vi "S2C_M2p5942_Proc_CallAcquire.vi"(7 "Command":string, 8 "Error In":errorcluster, 11 "Data":T1) -> (0 "Error Out":errorcluster)   [LabVIEW 2024]
uses:
  S2C_M2p5942_Proc_Globals.vi
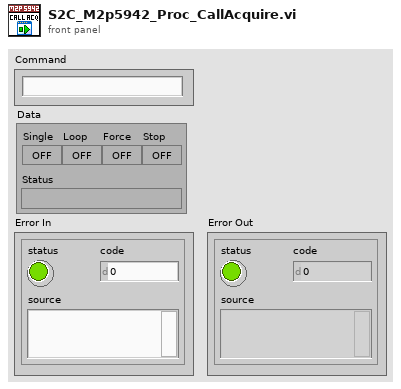
[diagram p1: front panel]
types:
  T1 = cluster{"Single":bool, "Loop":bool, "Force":bool, "Status":string, "Stop":bool}
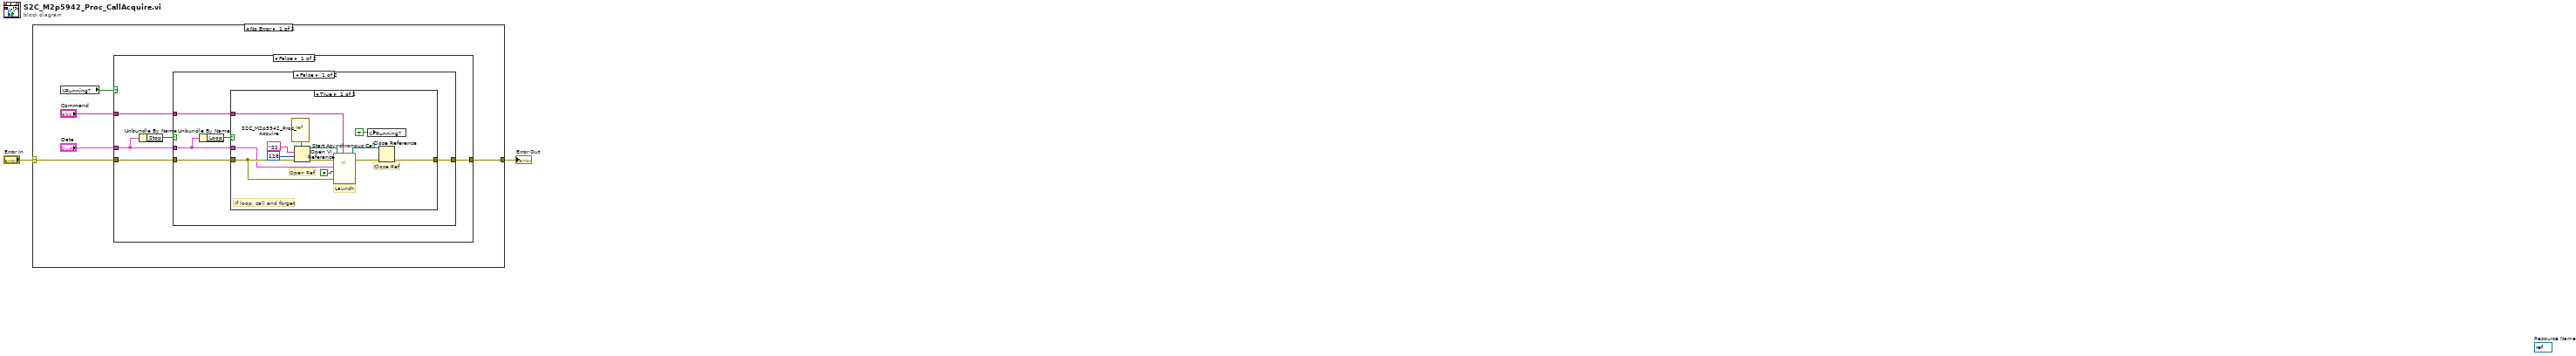
[diagram p0: block diagram]
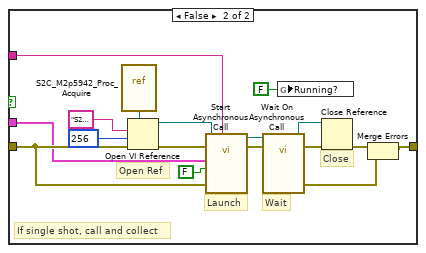
[diagram p2: hidden frame]
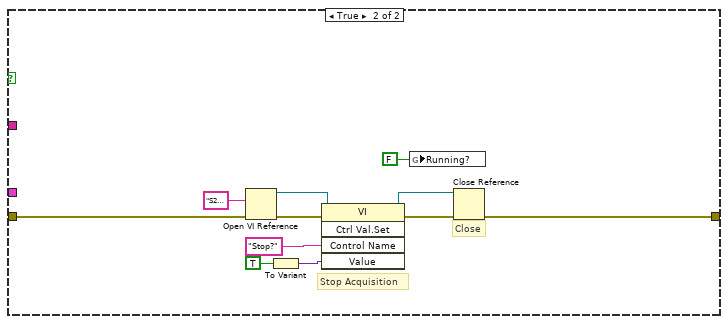
[diagram p4: hidden frame]
diagram:
  (unwired) refnum<visa-resource-name> refnum  # Resource Name
  n1 = case shown="No Error" "Error In" {
    selector: "Error In" -> [w7 w60]
    tunnel: [w6 w60] -> w1
    frame No Error {
      n2 = global read "S2C_M2p5942_Proc_Globals.vi" "Running?"() -> (w3:bool)
      n3 = case shown="False" w3 {
        tunnel: w7 -> [w12 w59]
        tunnel: [w11 w49] -> w6
        tunnel: "Command" -> [w10 _]
        tunnel: "Data" -> [w9 _]
        frame False {
          n4 = Unbundle By Name(w9) -> ("Stop"=w8:bool)
          n5 = case shown="False" w8 {
            tunnel: w12 -> [w17 w48]
            tunnel: [w16 w48] -> w11
            tunnel: w10 -> [w15 _]
            tunnel: w9 -> [w13 _]
            frame False {
              n6 = Unbundle By Name(w13) -> ("Loop"=w14:bool)
              n7 = case shown="True" w14 {
                tunnel: w15 -> [w24 w41]
                tunnel: w17 -> [w23 w40]
                tunnel: [w22 w35] -> w16
                tunnel: w13 -> [w21 w39]
                frame True {
                  # "If loop, call and forget"
                  # "Close Ref"
                  # "Launch"
                  # "Open Ref"
                  n8 = vi-ref "S2C_M2p5942_Proc_Acquire.vi"() -> (w29:refnum<vi>)
                  n9 = Open VI Reference(type specifier VI Refnum (for type only)=w29, vi path="S2C_M2p5942_Proc_Acquire.vi", options=128, error in (no error)=w23) -> (vi reference=w27:refnum<vi>, error out=w28:errorcluster)  [unwired: 2 in]
                  n10 = call-by-ref "Start Asynchronous Call"(reference=w27, error in=w28, "Command"=w24, "Error In"=w23, "Stop?"=FALSE, "Data"=w21) -> (reference out=w20:refnum<vi>, error out=w30:errorcluster)  [unwired: 7 in, 1 out]
                  n11 = global write "S2C_M2p5942_Proc_Globals.vi" "Running?"(TRUE ("Running?")) -> ()
                  n12 = Close Reference(reference=w20, error in (no error)=w30) -> (error out=w22:errorcluster)
                }
                frame False {
                  # "If single shot, call and collect"
                  # "Wait"
                  # "Close"
                  # "Launch"
                  # "Open Ref"
                  n13 = vi-ref "S2C_M2p5942_Proc_Acquire.vi"() -> (w46:refnum<vi>)
                  n14 = Open VI Reference(type specifier VI Refnum (for type only)=w46, vi path="S2C_M2p5942_Proc_Acquire.vi", options=256, error in (no error)=w40) -> (vi reference=w44:refnum<vi>, error out=w45:errorcluster)  [unwired: 2 in]
                  n15 = call-by-ref "Start Asynchronous Call"(reference=w44, error in=w45, "Command"=w41, "Error In"=w40, "Stop?"=FALSE, "Data"=w39) -> (reference out=w38:refnum<vi>, error out=w47:errorcluster)  [unwired: 7 in, 1 out]
                  n16 = call-by-ref "Wait On Asynchronous Call"(reference=w38, error in=w47) -> (reference out=w36:refnum<vi>, error out=w37:errorcluster, "Error Out"=w33:errorcluster)  [unwired: 11 in]
                  n17 = global write "S2C_M2p5942_Proc_Globals.vi" "Running?"(FALSE ("Running?")) -> ()
                  n18 = Close Reference(reference=w36, error in (no error)=w37) -> (error out=w34:errorcluster)
                  n19 = Merge Errors(w34, w33) -> (w35:errorcluster)
                }
              }
            }
            frame True {
            }
          }
        }
        frame True {
          # "Stop Acquisition"
          # "Close"
          n20 = Open VI Reference(vi path="S2C_M2p5942_Proc_Acquire.vi", error in (no error)=w59) -> (vi reference=w55:refnum<vi>, error out=w56:errorcluster)  [unwired: 4 in]
          n21 = To Variant(anything=TRUE) -> (Variant=w53:variant)
          n22 = invoke class="VI" method="Ctrl Val.Set"(reference=w55, error in=w56, "Control Name"="Stop?", "Value"=w53) -> (reference out=w50:refnum<vi>, error out=w51:errorcluster)  [unwired: 1 in, 3 out]
          n23 = global write "S2C_M2p5942_Proc_Globals.vi" "Running?"(FALSE ("Running?")) -> ()
          n24 = Close Reference(reference=w50, error in (no error)=w51) -> (error out=w49:errorcluster)
        }
      }
    }
    frame Error {
    }
  }
  "Error Out" <- w1
